vi "Biometry Average2String General.vi"(8 "error in (no error)":errorcluster caption="错误输入（无错误）", 9 "Biometry Average Standard Deviation":T1, 10 "Biometry Average State":T2, 11 "Biometry Average Parameter":T3) -> (0 "error out":errorcluster caption="错误输出", 2 "Data Output":string[][](array[string]))   [LabVIEW 2015, in "Utility VIs.lvlib"]
doc: "该模板用于创建子VI。"
uses:
  Utility VIs.lvlib
  Database Processing/Support/Table/Biometry Average Parameter.ctl
  Database Processing/Support/Table/Biometry Average State.ctl
  Database Processing/Support/Table/Biometry Average Standard Deviation.ctl
  Database Processing/Database Processing.lvlib
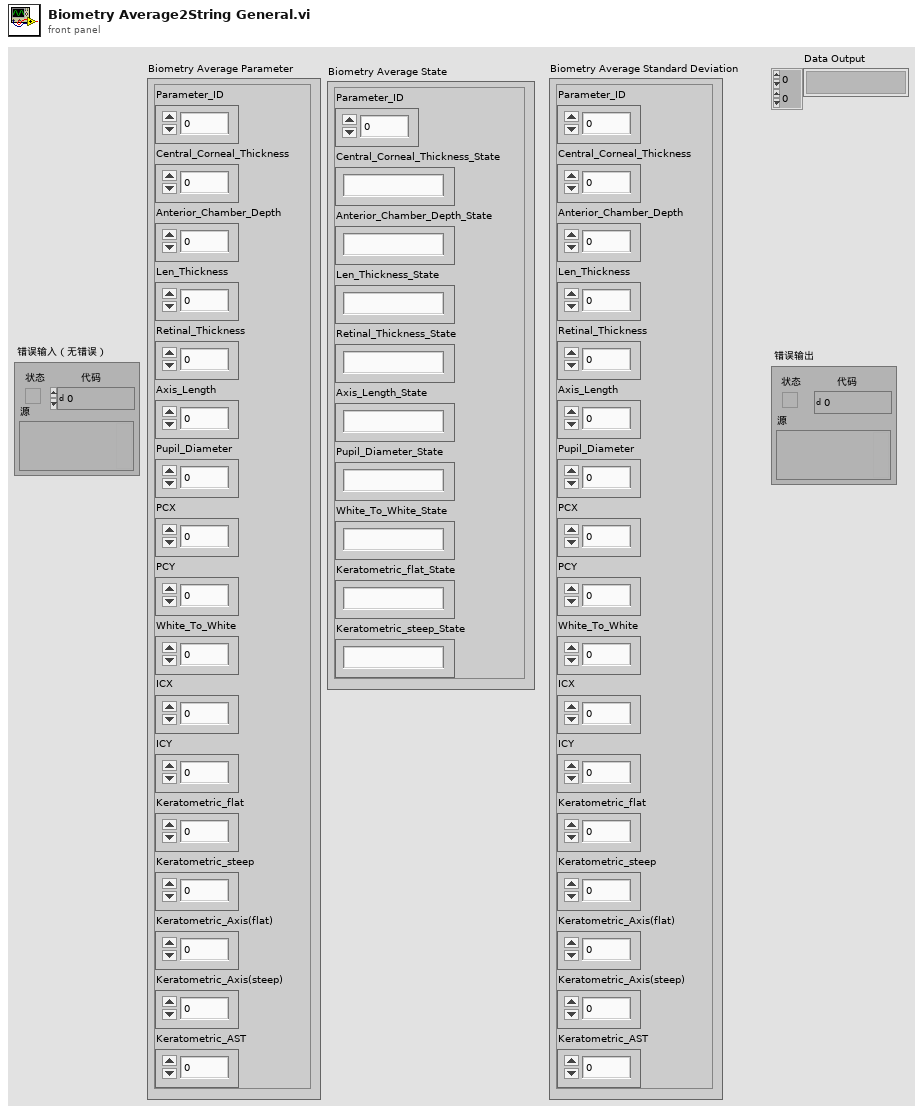
[diagram p1: front panel]
types:
  T1 = typedef "Database Processing.lvlib/Biometry Average Standard Deviation.ctl" = cluster{"Parameter_ID":i64, "Central_Corneal_Thickness":sgl, "Anterior_Chamber_Depth":sgl, "Len_Thickness":sgl, "Retinal_Thickness":sgl, "Axis_Length":sgl, "Pupil_Diameter":sgl, "PCX":sgl, "PCY":sgl, "White_To_White":sgl, "ICX":sgl, "ICY":sgl, "Keratometric_flat":sgl, "Keratometric_steep":sgl, "Keratometric_Axis(flat)":sgl, "Keratometric_Axis(steep)":sgl, "Keratometric_AST":sgl}
  T2 = typedef "Database Processing.lvlib/Biometry Average State.ctl" = cluster{"Parameter_ID":i64, "Central_Corneal_Thickness_State":string, "Anterior_Chamber_Depth_State":string, "Len_Thickness_State":string, "Retinal_Thickness_State":string, "Axis_Length_State":string, "Pupil_Diameter_State":string, "White_To_White_State":string, "Keratometric_flat_State":string, "Keratometric_steep_State":string}
  T3 = typedef "Database Processing.lvlib/Biometry Average Parameter.ctl" = cluster{"Parameter_ID":i64, "Central_Corneal_Thickness":sgl, "Anterior_Chamber_Depth":sgl, "Len_Thickness":sgl, "Retinal_Thickness":sgl, "Axis_Length":sgl, "Pupil_Diameter":sgl, "PCX":sgl, "PCY":sgl, "White_To_White":sgl, "ICX":sgl, "ICY":sgl, "Keratometric_flat":sgl, "Keratometric_steep":sgl, "Keratometric_Axis(flat)":sgl, "Keratometric_Axis(steep)":sgl, "Keratometric_AST":sgl}
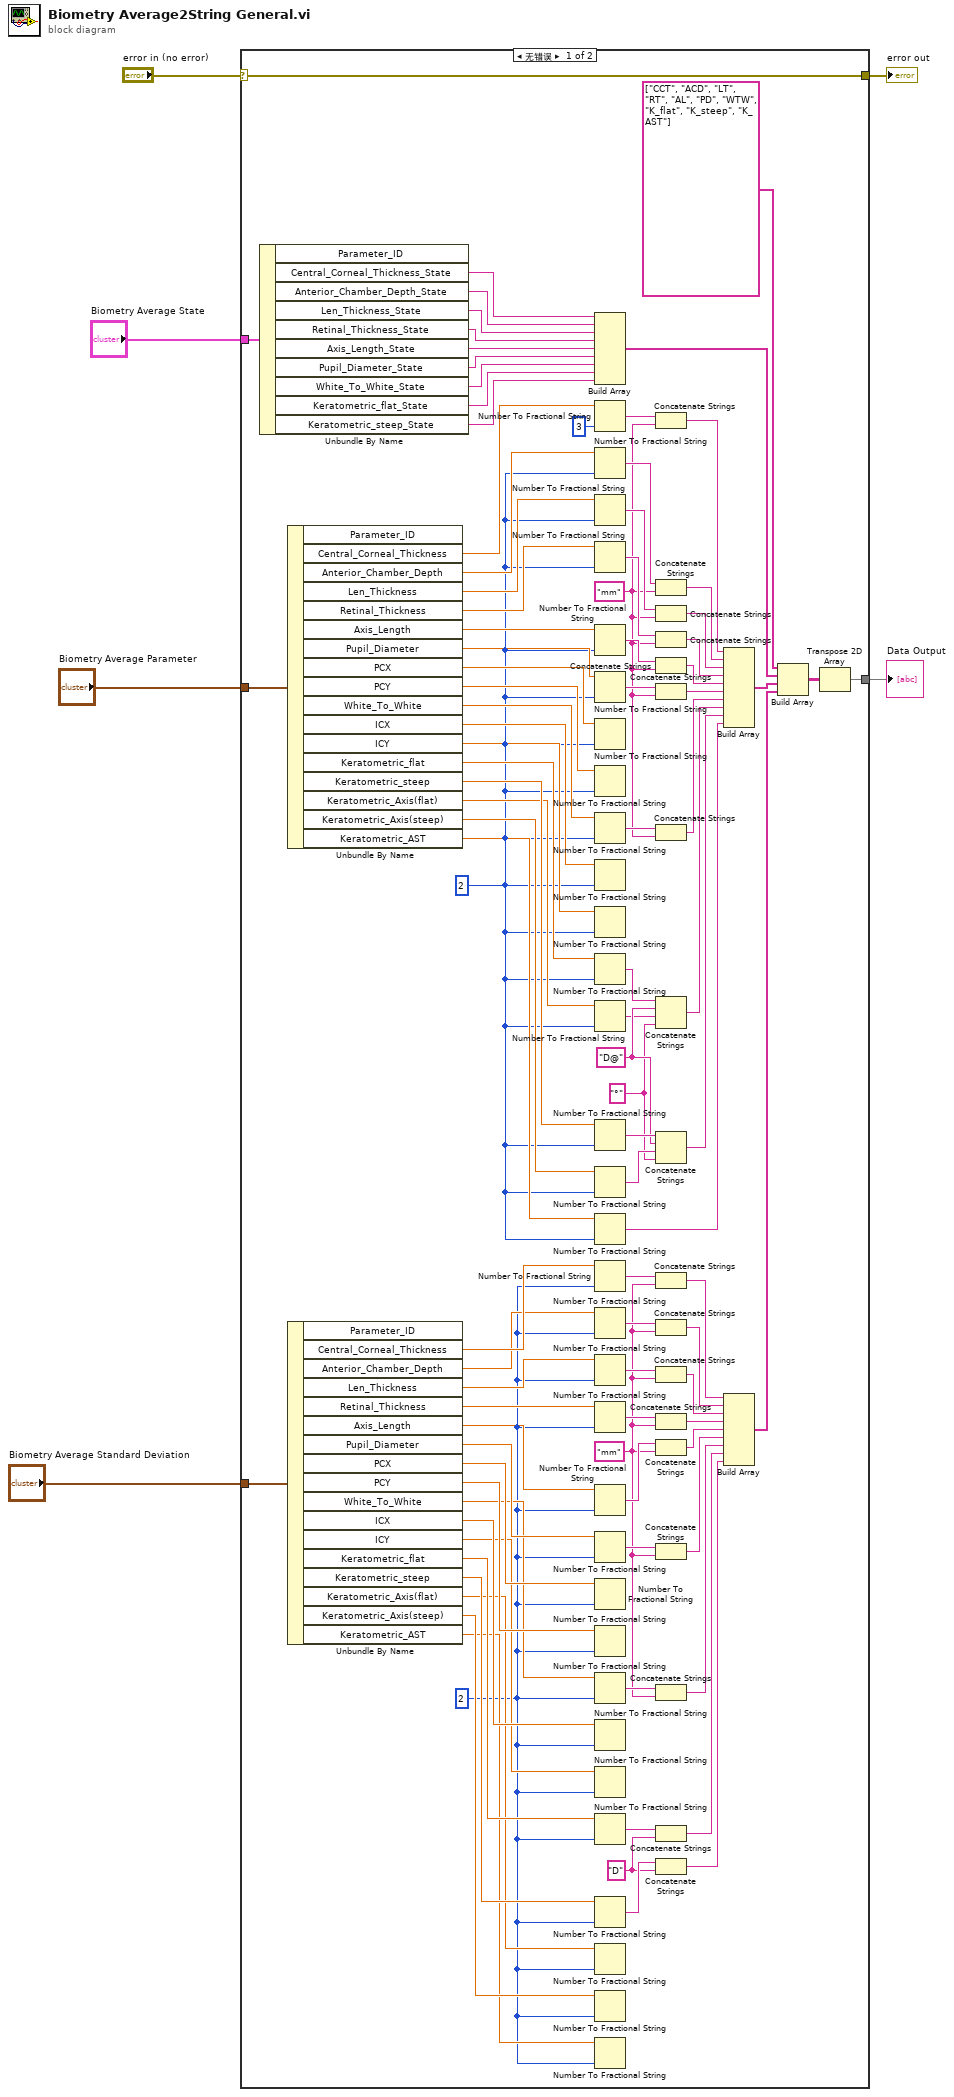
[diagram p0: block diagram]
diagram:
  n1 = case shown="无错误" "error in (no error)" {
    selector: "error in (no error)" -> [w12 w105]
    tunnel: [w12 w105] -> w5
    tunnel: "Biometry Average Parameter" -> [w104 _]
    tunnel: "Biometry Average Standard Deviation" -> [w103 _]
    tunnel: "Biometry Average State" -> [w102 _]
    tunnel: [w9 _] -> w1
    frame No Error {
      w44 = "D" ("字符串")
      w43 = "mm" ("字符串")
      w47 = i16 2 ("精度(6)")
      w57 = "°" ("字符串")
      w63 = "D@" ("字符串")
      w64 = "mm" ("字符串")
      w59 = i16 2 ("精度(6)")
      n2 = Unbundle By Name(w102) -> ("Central_Corneal_Thickness_State"=w42:string, "Anterior_Chamber_Depth_State"=w41:string, "Len_Thickness_State"=w40:string, "Retinal_Thickness_State"=w39:string, "Axis_Length_State"=w38:string, "Pupil_Diameter_State"=w37:string, "White_To_White_State"=w36:string, "Keratometric_flat_State"=w35:string, "Keratometric_steep_State"=w34:string)  [unwired: 1 out]
      n3 = Unbundle By Name(w104) -> ("Central_Corneal_Thickness"=w101:sgl, "Anterior_Chamber_Depth"=w100:sgl, "Len_Thickness"=w99:sgl, "Retinal_Thickness"=w98:sgl, "Axis_Length"=w97:sgl, "Pupil_Diameter"=w96:sgl, "PCX"=w95:sgl, "PCY"=w94:sgl, "White_To_White"=w93:sgl, "ICX"=w92:sgl, "ICY"=w91:sgl, "Keratometric_flat"=w90:sgl, "Keratometric_steep"=w89:sgl, "Keratometric_Axis(flat)"=w88:sgl, "Keratometric_Axis(steep)"=w61:sgl, "Keratometric_AST"=w60:sgl)  [unwired: 1 out]
      n4 = Unbundle By Name(w103) -> ("Central_Corneal_Thickness"=w87:sgl, "Anterior_Chamber_Depth"=w86:sgl, "Len_Thickness"=w85:sgl, "Retinal_Thickness"=w84:sgl, "Axis_Length"=w83:sgl, "Pupil_Diameter"=w82:sgl, "PCX"=w81:sgl, "PCY"=w80:sgl, "White_To_White"=w79:sgl, "ICX"=w78:sgl, "ICY"=w77:sgl, "Keratometric_flat"=w76:sgl, "Keratometric_steep"=w75:sgl, "Keratometric_Axis(flat)"=w74:sgl, "Keratometric_Axis(steep)"=w49:sgl, "Keratometric_AST"=w48:sgl)  [unwired: 1 out]
      n5 = Build Array(w42, w41, w40, w39, w38, w37, w36, w35, w34) -> (w15:string[])
      n6 = Number To Fractional String(number=w101, precision (6)=i16 3 ("精度(6)")) -> (F-format string=w73:string)  [unwired: 2 in]
      n7 = Number To Fractional String(number=w100, precision (6)=w59) -> (F-format string=w72:string)  [unwired: 2 in]
      n8 = Number To Fractional String(number=w99, precision (6)=w59) -> (F-format string=w71:string)  [unwired: 2 in]
      n9 = Number To Fractional String(number=w98, precision (6)=w59) -> (F-format string=w70:string)  [unwired: 2 in]
      n10 = Number To Fractional String(number=w97, precision (6)=w59) -> (F-format string=w69:string)  [unwired: 2 in]
      n11 = Number To Fractional String(number=w96, precision (6)=w59) -> (F-format string=w68:string)  [unwired: 2 in]
      n12 = Number To Fractional String(number=w95, precision (6)=w59) -> ()  [unwired: 2 in, 1 out]
      n13 = Number To Fractional String(number=w94, precision (6)=w59) -> ()  [unwired: 2 in, 1 out]
      n14 = Number To Fractional String(number=w93, precision (6)=w59) -> (F-format string=w67:string)  [unwired: 2 in]
      n15 = Number To Fractional String(number=w92, precision (6)=w59) -> ()  [unwired: 2 in, 1 out]
      n16 = Number To Fractional String(number=w91, precision (6)=w59) -> ()  [unwired: 2 in, 1 out]
      n17 = Number To Fractional String(number=w90, precision (6)=w59) -> (F-format string=w66:string)  [unwired: 2 in]
      n18 = Number To Fractional String(number=w88, precision (6)=w59) -> (F-format string=w62:string)  [unwired: 2 in]
      n19 = Number To Fractional String(number=w89, precision (6)=w59) -> (F-format string=w65:string)  [unwired: 2 in]
      n20 = Number To Fractional String(number=w61, precision (6)=w59) -> (F-format string=w58:string)  [unwired: 2 in]
      n21 = Number To Fractional String(number=w60, precision (6)=w59) -> (F-format string=w7:string)  [unwired: 2 in]
      n22 = Number To Fractional String(number=w87, precision (6)=w47) -> (F-format string=w56:string)  [unwired: 2 in]
      n23 = Number To Fractional String(number=w86, precision (6)=w47) -> (F-format string=w55:string)  [unwired: 2 in]
      n24 = Number To Fractional String(number=w85, precision (6)=w47) -> (F-format string=w54:string)  [unwired: 2 in]
      n25 = Number To Fractional String(number=w84, precision (6)=w47) -> (F-format string=w53:string)  [unwired: 2 in]
      n26 = Number To Fractional String(number=w83, precision (6)=w47) -> (F-format string=w52:string)  [unwired: 2 in]
      n27 = Number To Fractional String(number=w82, precision (6)=w47) -> (F-format string=w51:string)  [unwired: 2 in]
      n28 = Number To Fractional String(number=w81, precision (6)=w47) -> ()  [unwired: 2 in, 1 out]
      n29 = Number To Fractional String(number=w80, precision (6)=w47) -> ()  [unwired: 2 in, 1 out]
      n30 = Number To Fractional String(number=w79, precision (6)=w47) -> (F-format string=w50:string)  [unwired: 2 in]
      n31 = Number To Fractional String(number=w78, precision (6)=w47) -> ()  [unwired: 2 in, 1 out]
      n32 = Number To Fractional String(number=w77, precision (6)=w47) -> ()  [unwired: 2 in, 1 out]
      n33 = Number To Fractional String(number=w76, precision (6)=w47) -> (F-format string=w46:string)  [unwired: 2 in]
      n34 = Number To Fractional String(number=w75, precision (6)=w47) -> (F-format string=w45:string)  [unwired: 2 in]
      n35 = Number To Fractional String(number=w74, precision (6)=w47) -> ()  [unwired: 2 in, 1 out]
      n36 = Number To Fractional String(number=w49, precision (6)=w47) -> ()  [unwired: 2 in, 1 out]
      n37 = Number To Fractional String(number=w48, precision (6)=w47) -> ()  [unwired: 2 in, 1 out]
      n38 = Concatenate Strings(w73, w64) -> (w33:string)
      n39 = Concatenate Strings(w72, w64) -> (w32:string)
      n40 = Concatenate Strings(w71, w64) -> (w31:string)
      n41 = Concatenate Strings(w70, w64) -> (w30:string)
      n42 = Concatenate Strings(w69, w64) -> (w29:string)
      n43 = Concatenate Strings(w68, w64) -> (w28:string)
      n44 = Concatenate Strings(w67, w64) -> (w27:string)
      n45 = Concatenate Strings(w66, w63, w62, w57) -> (w26:string)
      n46 = Concatenate Strings(w65, w63, w58, w57) -> (w25:string)
      n47 = Concatenate Strings(w56, w43) -> (w24:string)
      n48 = Concatenate Strings(w55, w43) -> (w23:string)
      n49 = Concatenate Strings(w54, w43) -> (w22:string)
      n50 = Concatenate Strings(w53, w43) -> (w21:string)
      n51 = Concatenate Strings(w52, w43) -> (w20:string)
      n52 = Concatenate Strings(w51, w43) -> (w19:string)
      n53 = Concatenate Strings(w50, w43) -> (w18:string)
      n54 = Concatenate Strings(w46, w44) -> (w17:string)
      n55 = Concatenate Strings(w45, w44) -> (w16:string)
      n56 = Build Array(w33, w32, w31, w30, w29, w28, w27, w26, w25, w7) -> (w13:string[])
      n57 = Build Array(w24, w23, w22, w21, w20, w19, w18, w17, w16) -> (w14:string[])
      n58 = Build Array(string[] ["CCT", "ACD", "LT", "RT", "AL", "PD", "WTW", "K_flat", "K_steep", "K_AST"] ("元素"), w15, w13, w14) -> (w10:string[][])
      n59 = Transpose 2D Array(2D array=w10) -> (transposed array=w9:string[][])
    }
    frame Error {
    }
  }
  "error out" <- w5
  "Data Output" <- w1
